vi "GetType.vi"(8 "error in (no error)":errorcluster, 11 "Write Polling Iterations Msg":refnum<class "Polling Iterations Msg.lvclass">) -> (0 "error out":errorcluster, 2 "Data Sample":variant, 3 "Write Polling Iterations Msg":refnum<class "Polling Iterations Msg.lvclass">)   [LabVIEW 2016, in "CS++BaseActor.lvlib" / "Polling Iterations Msg.lvclass"]
uses:
  Polling Iterations Msg.lvclass
  Polling Iterations Msg.lvclass/Polling Iterations Msg.ctl
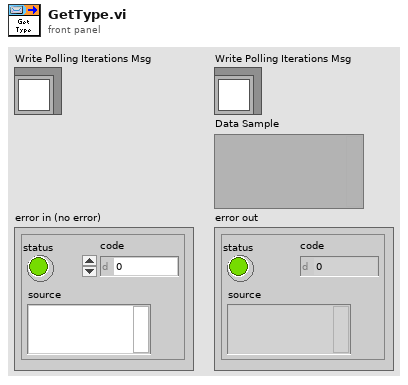
[diagram p1: front panel]
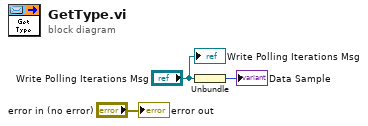
[diagram p0: block diagram]
diagram:
  n1 = Unbundle("Write Polling Iterations Msg") -> (→"Data Sample":u32)
  "error out" <- "error in (no error)"
  "Write Polling Iterations Msg" <- "Write Polling Iterations Msg"
